vi "Kaelus PIM Measure.vi"(6 "Legacy?":bool, 8 "error in (no error)":errorcluster) -> (0 "error out":errorcluster, 3 "Measurement Results":T1 {"IMPower_dBc(s)" format="%.2f"; "TxFreqs" format="%.2f"; "IMFreq(s)" format="%.2f"; "IMPower(s)" format="%.2f"; "TxPower" format="%.2f"})   [LabVIEW 2011]
uses:
  PIM Results.ctl
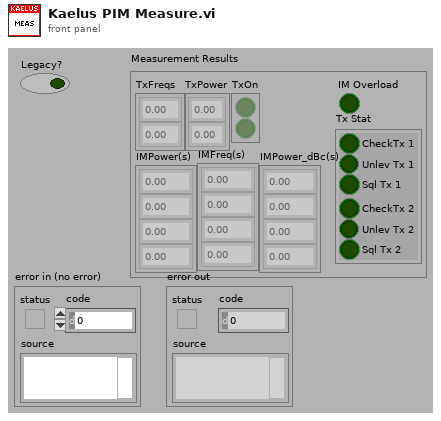
[diagram p1: front panel]
types:
  T1 = typedef "PIM Results.ctl" = cluster{"TxFreqs":dbl[], "TxPower":dbl[], "TxOn":bool[], "IMPower(s)":dbl[], "IMFreq(s)":dbl[], "Tx Stat":cluster{"CheckTx 1":bool, "Unlev Tx 1":bool, "Sql Tx 1":bool, "CheckTx 2":bool, "Unlev Tx 2":bool, "Sql Tx 2":bool}, "IM Overload":bool, "IMPower_dBc(s)":dbl[]}
  T2 = typedef "PIM.API.Command.Unique.ctl" = cluster{"#attributes":cluster{"Action":string}, "Double":dbl[], "Integer":i32[], "Boolean":bool[], "String":string[]}
  T3 = typedef "PIM.API.Response.Unique.ctl" = cluster{"#attributes":cluster{"Action":string, "Units":string}, "Double":dbl[], "Integer":i32[], "Boolean":bool[], "String":string[], "Sample":T4[], "Status":cluster{"#attributes":cluster{"Error":bool, "Code":i32}, "Message":string}[]}
  T4 = typedef "PIM.API.Response.Samples.ctl" = cluster{"TX1":cluster{"#attributes":cluster{"Frequency":dbl, "Power_dBm":dbl, "Power_Watts":dbl, "CheckTx":bool, "Unleveled":bool, "Squelched":bool, "Temperature":dbl, "ToneOn":bool}}, "TX2":cluster{"#attributes":cluster{"Frequency":dbl, "Power_dBm":dbl, "Power_Watts":dbl, "CheckTx":bool, "Unleveled":bool, "Squelched":bool, "Temperature":dbl, "ToneOn":bool}}, "IM":cluster{"#attributes":cluster{"Frequency":dbl, "Power_dBm":dbl, "PeakPower_dBm":dbl, "Power_dBc":dbl, "PeakPower_dBc":dbl, "IM_Order":u8, "IM Overload":bool}}[], "#attributes":cluster{"Count":u32, "Total":u32, "Finished?":bool, "Sweep Leg":T5, "F1":dbl, "F2":dbl, "FStep":dbl}}
  T5 = typedef "iQA Sweep Behavior.ctl" = enum16{"F2Down", "F1Up", "RxMultiIM"}
  T6 = cluster{"Boolean[0]":bool, "Boolean[1]":bool, "Boolean[2]":bool, "Boolean[3]":bool, "Boolean[4]":bool, "Boolean[5]":bool}
  T7 = cluster{"[0]":bool, "[1]":bool, "[2]":bool, "[3]":bool, "[4]":bool, "[5]":bool}
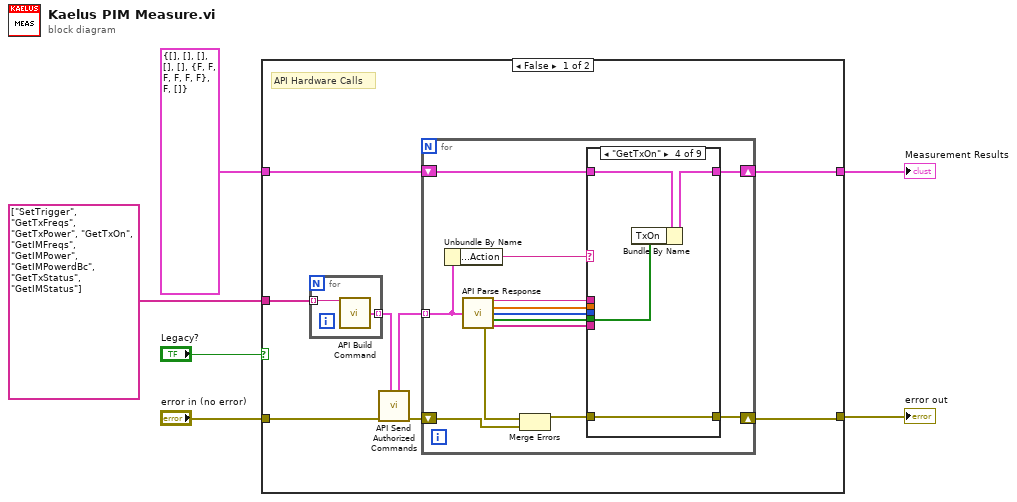
[diagram p0: block diagram]
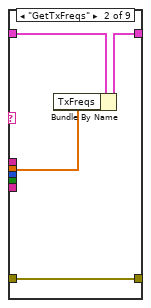
[diagram p3: hidden frame]
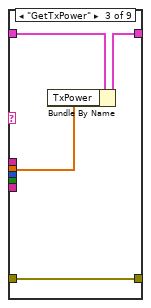
[diagram p4: hidden frame]
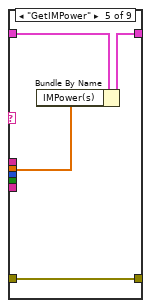
[diagram p5: hidden frame]
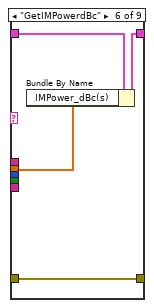
[diagram p6: hidden frame]
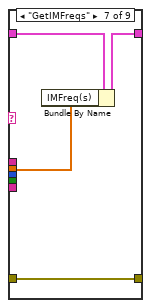
[diagram p7: hidden frame]
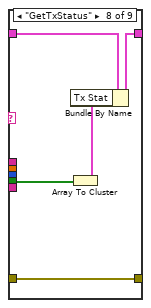
[diagram p8: hidden frame]
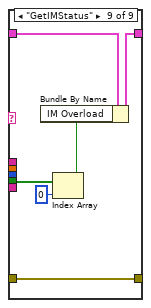
[diagram p9: hidden frame]
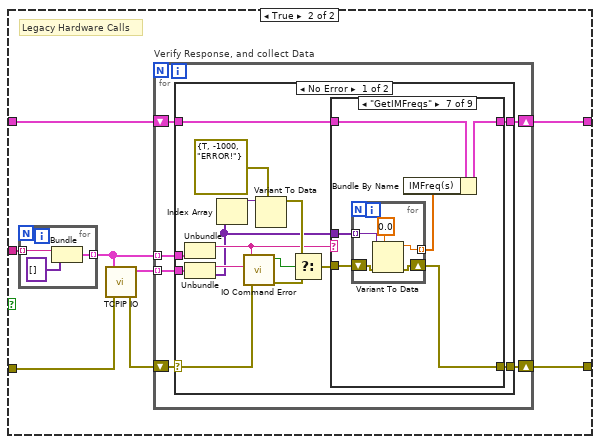
[diagram p10: hidden frame]
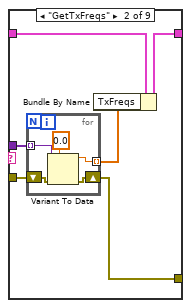
[diagram p12: hidden frame]
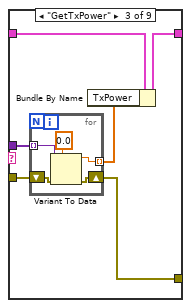
[diagram p13: hidden frame]
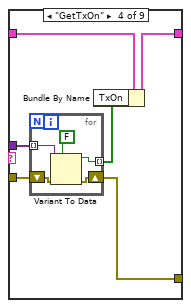
[diagram p14: hidden frame]
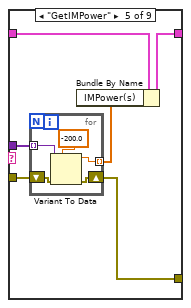
[diagram p15: hidden frame]
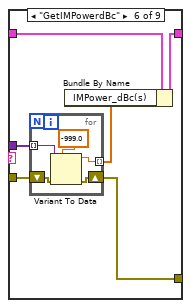
[diagram p16: hidden frame]
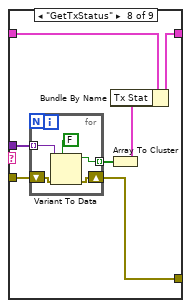
[diagram p17: hidden frame]
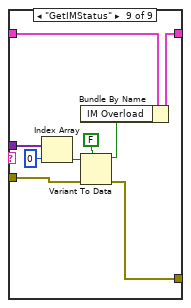
[diagram p18: hidden frame]
diagram:
  n1 = case shown="False" "Legacy?" {
    tunnel: "error in (no error)" -> [w12 w74]
    tunnel: T1 {"TxFreqs"=[], "TxPower"=[], "TxOn"=[], "IMPower(s)"=[], "IMFreq(s)"=[], "Tx Stat"={"CheckTx 1"=FALSE, "Unlev Tx 1"=FALSE, "Sql Tx 1"=FALSE, "CheckTx 2"=FALSE, "Unlev Tx 2"=FALSE, "Sql Tx 2"=FALSE}, "IM Overload"=FALSE, "IMPower_dBc(s)"=[]} ("Measurement Results") -> [w9 w70]
    tunnel: [w7 w69] -> w4
    tunnel: [w8 w68] -> w1
    tunnel: string[] ["SetTrigger", "GetTxFreqs", "GetTxPower", "GetTxOn", "GetIMFreqs", "GetIMPower", "GetIMPowerdBc", "GetTxStatus", "GetIMStatus"] -> [w14 w67]
    frame False {
      # "API Hardware Calls"
      n2 = for {
        tunnel: w14 -> [w66] mode=indexing
        tunnel: [w65] -> w13 mode=indexing
        n3 = call "API Build Command.vi"("Action"=w66) -> ("PIM.API.Command.Unique"=w65:T2)  [unwired: 14 in]
      }
      n4 = call "API Send Authorized Commands.vi"("Commands"=w13, "error in (no error)"=w12) -> ("error out"=w11:errorcluster, "Responses"=w10:T3[])  [unwired: 7 in, 1 out]
      n5 = for {
        shift-right: [w19] -> w8
        shift-left: w11 -> [w17]
        tunnel: w10 -> [w25] mode=indexing
        shift-right: [w15] -> w7
        shift-left: w9 -> [w26]
        n6 = Unbundle By Name(w25) -> ("#attributes.Action"=w27:string)
        n7 = call "API Parse Response.vi"("PIM.API.Response.Unique"=w25) -> ("Action"=w24:string, "Double"=w23:dbl[], "Integer"=w22:i32[], "Boolean"=w21:bool[], "error out"=w18:errorcluster, "String"=w20:string[])  [unwired: 8 in, 1 out]
        n8 = Merge Errors(w18, w17) -> (w16:errorcluster)
        n9 = case shown="\"GetTxOn\"" w27 {
          tunnel: w26 -> [w29 w33 w37 w41 w45 w49 w53 w58 w64]
          tunnel: [w29 w32 w36 w40 w44 w48 w52 w57 w63] -> w15
          tunnel: [w28 w30 w34 w38 w42 w46 w51 w55 w59] -> w19
          tunnel: w24 -> [_ _ _ _ _ _ _ _ _]
          tunnel: w23 -> [_ w31 w35 _ w43 w47 w50 _ _]
          tunnel: w22 -> [_ _ _ _ _ _ _ _ _]
          tunnel: w21 -> [_ _ _ w39 _ _ _ w54 w61]
          tunnel: w20 -> [_ _ _ _ _ _ _ _ _]
          tunnel: w16 -> [w28 w30 w34 w38 w42 w46 w51 w55 w59]
          frame "SetTrigger", Default {
            # "No Data to be set here"
          }
          frame "GetTxFreqs" {
            n10 = Bundle By Name(cluster=w33, "TxFreqs"=w31) -> (w32:T1)
          }
          frame "GetTxPower" {
            n11 = Bundle By Name(cluster=w37, "TxPower"=w35) -> (w36:T1)
          }
          frame "GetTxOn" {
            n12 = Bundle By Name(cluster=w41, "TxOn"=w39) -> (w40:T1)
          }
          frame "GetIMPower" {
            n13 = Bundle By Name(cluster=w45, "IMPower(s)"=w43) -> (w44:T1)
          }
          frame "GetIMPowerdBc" {
            n14 = Bundle By Name(cluster=w49, "IMPower_dBc(s)"=w47) -> (w48:T1)
          }
          frame "GetIMFreqs" {
            n15 = Bundle By Name(cluster=w53, "IMFreq(s)"=w50) -> (w52:T1)
          }
          frame "GetTxStatus" {
            n16 = Array To Cluster(array=w54) -> (cluster=w56:T6)
            n17 = Bundle By Name(cluster=w58, "Tx Stat"=w56) -> (w57:T1)
          }
          frame "GetIMStatus" {
            n18 = Index Array(array=w61, index=0) -> (element=w60:bool)
            n19 = Bundle By Name(cluster=w64, "IM Overload"=w60) -> (w63:T1)
          }
        }
      }
    }
    frame True {
      # "Legacy Hardware Calls"
      n20 = for {
        tunnel: w67 -> [w189] mode=indexing
        tunnel: [w187] -> w73 mode=indexing
        n21 = Bundle(w189, variant[] []) -> (w187:cluster{string, variant[]})  [unwired: 1 out]
      }
      n22 = call "TCPIP IO.vi"("error in (no error)"=w74, "Commands"=w73) -> ("error out"=w71:errorcluster, "Responses"=w72:cluster{string, variant[]}[])  [unwired: 1 in, 3 out]
      n23 = for "Verify Response, and collect Data" {
        tunnel: w72 -> [w79] mode=indexing
        tunnel: w73 -> [w80] mode=indexing
        shift-right: [w76] -> w68
        shift-left: w71 -> [w75]
        shift-right: [w77] -> w69
        shift-left: w70 -> [w78]
        n24 = case shown="No Error" w75 {
          selector: w75 -> [w81 w185]
          tunnel: w80 -> [w95 _]
          tunnel: w79 -> [w94 _]
          tunnel: w78 -> [w86 w186]
          tunnel: [w85 w186] -> w77
          tunnel: [w82 w185] -> w76
          frame No Error {
            n25 = Unbundle(w95) -> (w87:string)  [unwired: 1 out]
            n26 = Unbundle(w94) -> (w93:string, w84:variant[])
            n27 = Index Array(array=w84) -> (element=w91:variant)  [unwired: 1 in]
            n28 = call "IO Command Error.vi"("error in (no error)"=w81, "Command Returned (\"\")"=w93, "Command Sent (\"\")"=w87) -> ("error out"=w88:errorcluster, "HW ERR?"=w90:bool)  [unwired: 3 out]
            n29 = Variant To Data(type=errorcluster {"status"=TRUE, "code"=-1000, "source"="ERROR!"} ("error out"), Variant=w91) -> (data=w89:errorcluster)  [unwired: 1 in, 1 out]
            n30 = Select(t=w89, s=w90, f=w88) -> (s? t:f=w83:errorcluster)
            n31 = case shown="\"GetIMFreqs\"" w87 {
              tunnel: w86 -> [w97 w99 w111 w122 w133 w144 w155 w167 w182]
              tunnel: [w97 w98 w110 w121 w132 w143 w154 w166 w181] -> w85
              tunnel: w84 -> [_ w103 w114 w125 w136 w147 w158 w170 w178]
              tunnel: w83 -> [w96 w102 w113 w124 w135 w146 w157 w169 w184]
              tunnel: [w96 w101 w112 w123 w134 w145 w156 w168 w183] -> w82
              frame "SetTrigger", Default {
                # "No Data to be set here"
              }
              frame "GetTxFreqs" {
                n32 = for {
                  tunnel: w103 -> [w106] mode=indexing
                  shift-right: [w107] -> w101
                  shift-left: w102 -> [w108]
                  tunnel: [w105] -> w100 mode=indexing
                  n33 = Variant To Data(error in=w108, type=0.0, Variant=w106) -> (data=w105:dbl, error out=w107:errorcluster)
                }
                n34 = Bundle By Name(cluster=w99, "TxFreqs"=w100) -> (w98:T1)
              }
              frame "GetTxPower" {
                n35 = for {
                  tunnel: w114 -> [w117] mode=indexing
                  shift-right: [w118] -> w112
                  shift-left: w113 -> [w119]
                  tunnel: [w116] -> w109 mode=indexing
                  n36 = Variant To Data(error in=w119, type=0.0, Variant=w117) -> (data=w116:dbl, error out=w118:errorcluster)
                }
                n37 = Bundle By Name(cluster=w111, "TxPower"=w109) -> (w110:T1)
              }
              frame "GetTxOn" {
                n38 = for {
                  tunnel: w125 -> [w128] mode=indexing
                  shift-right: [w129] -> w123
                  shift-left: w124 -> [w130]
                  tunnel: [w127] -> w120 mode=indexing
                  n39 = Variant To Data(error in=w130, type=FALSE ("status"), Variant=w128) -> (data=w127:bool, error out=w129:errorcluster)
                }
                n40 = Bundle By Name(cluster=w122, "TxOn"=w120) -> (w121:T1)
              }
              frame "GetIMPower" {
                n41 = for {
                  tunnel: w136 -> [w139] mode=indexing
                  shift-right: [w140] -> w134
                  shift-left: w135 -> [w141]
                  tunnel: [w138] -> w131 mode=indexing
                  n42 = Variant To Data(error in=w141, type=-200.0, Variant=w139) -> (data=w138:dbl, error out=w140:errorcluster)
                }
                n43 = Bundle By Name(cluster=w133, "IMPower(s)"=w131) -> (w132:T1)
              }
              frame "GetIMPowerdBc" {
                n44 = for {
                  tunnel: w147 -> [w150] mode=indexing
                  shift-right: [w151] -> w145
                  shift-left: w146 -> [w152]
                  tunnel: [w149] -> w142 mode=indexing
                  n45 = Variant To Data(error in=w152, type=-999.0, Variant=w150) -> (data=w149:dbl, error out=w151:errorcluster)
                }
                n46 = Bundle By Name(cluster=w144, "IMPower_dBc(s)"=w142) -> (w143:T1)
              }
              frame "GetIMFreqs" {
                n47 = for {
                  tunnel: w158 -> [w161] mode=indexing
                  shift-right: [w162] -> w156
                  shift-left: w157 -> [w163]
                  tunnel: [w160] -> w153 mode=indexing
                  n48 = Variant To Data(error in=w163, type=0.0, Variant=w161) -> (data=w160:dbl, error out=w162:errorcluster)
                }
                n49 = Bundle By Name(cluster=w155, "IMFreq(s)"=w153) -> (w154:T1)
              }
              frame "GetTxStatus" {
                n50 = for {
                  tunnel: w170 -> [w173] mode=indexing
                  shift-right: [w174] -> w168
                  shift-left: w169 -> [w175]
                  tunnel: [w172] -> w165 mode=indexing
                  n51 = Variant To Data(error in=w175, type=FALSE ("status"), Variant=w173) -> (data=w172:bool, error out=w174:errorcluster)
                }
                n52 = Array To Cluster(array=w165) -> (cluster=w164:T7)
                n53 = Bundle By Name(cluster=w167, "Tx Stat"=w164) -> (w166:T1)
              }
              frame "GetIMStatus" {
                n54 = Index Array(array=w178, index=0) -> (element=w176:variant)
                n55 = Variant To Data(error in=w184, type=FALSE ("status"), Variant=w176) -> (data=w179:bool, error out=w183:errorcluster)
                n56 = Bundle By Name(cluster=w182, "IM Overload"=w179) -> (w181:T1)
              }
            }
          }
          frame Error {
          }
        }
      }
    }
  }
  "Measurement Results" <- w4
  "error out" <- w1
